vi "Quaternion_Get_Vect.vi"(11 "Quaternion":T1={"R"=1.0, "V"=[0.0, 0.0, 0.0]}) -> (3 "Vector":dbl[](array[numeric]))   [LabVIEW 2019, in "Trajectory_Library.lvlib"]
doc: "Get the Vector component of the Quaternion data cluster\n\nInput:\n - Quaternion -- Quaternion data cluster\n\nOutput:\n - Vector -- Vector component of the quaternion as an array."
uses:
  Trajectory_Library.lvlib
  QUATERNION.ctl
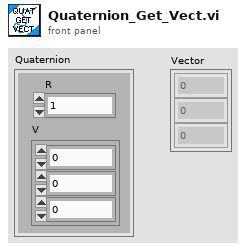
[diagram p1: front panel]
types:
  T1 = typedef "Trajectory_Library.lvlib/QUATERNION.ctl" = cluster{"R":dbl, "V":dbl[]}
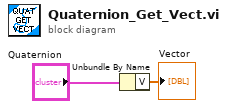
[diagram p0: block diagram]
diagram:
  n1 = Unbundle By Name("Quaternion") -> ("V"=→"Vector":dbl[])
